vi "Set Configuration.vi"(8 "error in (no error)":errorcluster, 11 "FPGA Addon Input in":refnum<class "FPGA Addon Input.lvclass">) -> (0 "error out":errorcluster, 3 "FPGA Addon Input out":refnum<class "FPGA Addon Input.lvclass">)   [LabVIEW 2015, in "FPGA Addon Input.lvclass"]
uses:
  FPGA Addon Input.lvclass
  IO Class/Classification.ctl
  Input Signal/Input Signal.lvclass
  IO Class/IO Class.lvclass
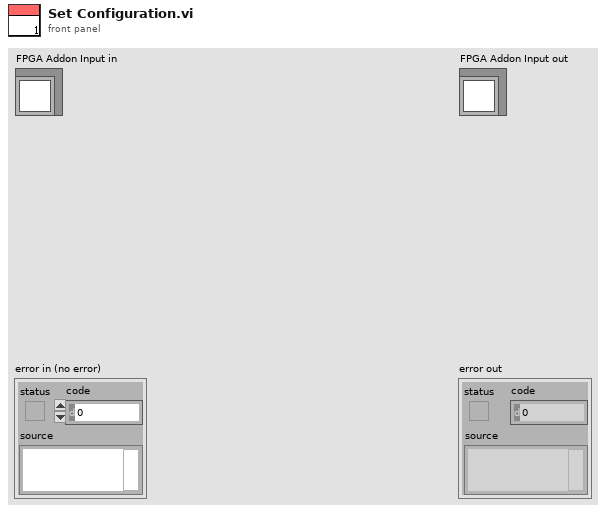
[diagram p1: front panel]
types:
  T1 = typedef "IO Class.lvclass/Classification.ctl" = cluster{"Classification":string}
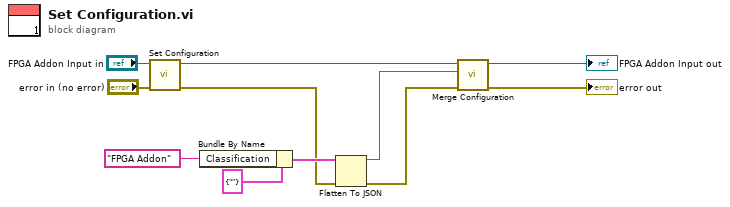
[diagram p0: block diagram]
diagram:
  n1 = call-parent "Set Configuration.vi"("error in (no error)"="error in (no error)", "Input Signal in"="FPGA Addon Input in") -> ("error out"=w6:errorcluster, "Input Signal out"=w5:refnum<class "FPGA Addon Input.lvclass">)  [unwired: 8 in]
  n2 = Bundle By Name(cluster=T1 {"Classification"=""} ("Classification"), "Classification"="FPGA Addon" ("Type")) -> (w8:T1)
  n3 = Flatten To JSON(anything=w8, error in (no error)=w6) -> (JSON string=w1:string, 11:w3:errorcluster)  [unwired: 1 in]
  n4 = call "Merge Configuration.vi"("error in (no error)"=w3, "Additional Configuration"=w1, "IO Class in"=w5) -> ("error out"=→"error out":errorcluster, "IO Class out"=→"FPGA Addon Input out":refnum<class "FPGA Addon Input.lvclass">)  [unwired: 7 in]
